vi "Test Draw Polylines ARGB.vi"(8 "error in (no error)":errorcluster, 11 "Test Case In":refnum<class "Image.lvclass">) -> (0 "error out":errorcluster, 3 "Test Case Out":refnum<class "Image.lvclass">)   [LabVIEW 2020, in "g_ar_toolkit.test.lvlib" / "Image.lvclass"]
uses:
  Image.lvclass
  C:/Program Files (x86)/National Instruments/LabVIEW 2020/vi.lib/Astemes/LUnit/Test Case.lvclass
  g_ar_toolkit.image/ARGB Colour.ctl
  g_ar_toolkit.common/Image Size (Integer).ctl
  g_ar_toolkit.common/Image Point (Integer).ctl
  <vilib>/Astemes/LUnit/Test Case.lvclass/Test Case.ctl
  g_ar_toolkit.image/CreateEmptyImageARGB.vi
  4993e8ee-a06a-463a-9684-69129f64d5ce.vi
  g_ar_toolkit.image/CreateEmptyImageARGB.vi/3321fa97-f432-4e1e-8db9-a0df79aed21b.vi
  g_ar_toolkit.image/DrawPolyLinesOnImageARGB.vi/f4fe866f-059f-471d-887d-2797bd4b3b13.vi
  g_ar_toolkit.image/DrawImageToPictureARGB.vi/8cd07b1b-062e-4fe4-9e87-2eb3dc89fe0e.vi
  <vilib>/Astemes/LUnit/Append Pass Result.vi
  <vilib>/Astemes/LUnit/Append Fail Result.vi
  <vilib>/Astemes/LUnit/Describe Comparison.vi
  <vilib>/Astemes/LUnit/Compare Variants.vi
  <vilib>/Astemes/LUnit/Run In UI.vi
  <vilib>/Utility/error.llb/Clear Errors.vi
  g_ar_toolkit.image/ARGBColourToU32.vi
  g_ar_toolkit.common/Module Path.vi
  <vilib>/Utility/error.llb/Error Cluster From Error Code.vi
  <vilib>/Astemes/LUnit/Describe Variant.vi
  Image.lvclass/Image.ctl
  g_ar_toolkit.image/g_ar_toolkit.image.lvlib
  g_ar_toolkit.common/g_ar_toolkit.common.lvlib
panel:
  out "Picture":picture
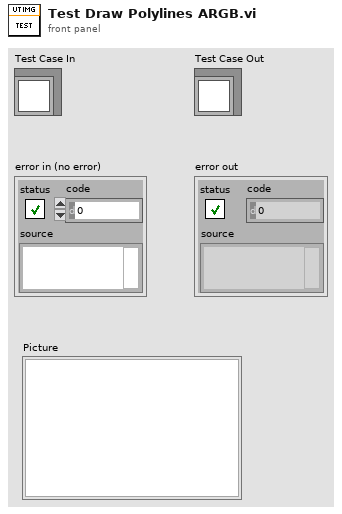
[diagram p1: front panel]
types:
  T1 = typedef "g_ar_toolkit.common.lvlib/Image Point (Integer).ctl" = cluster{"x":i32, "y":i32}
  T2 = typedef "g_ar_toolkit.image.lvlib/ARGB Colour.ctl" = cluster{"Alpha":u8, "RGB":u32}
  T3 = typedef "g_ar_toolkit.common.lvlib/Image Size (Integer).ctl" = cluster{"Width":u16, "Height":u16}
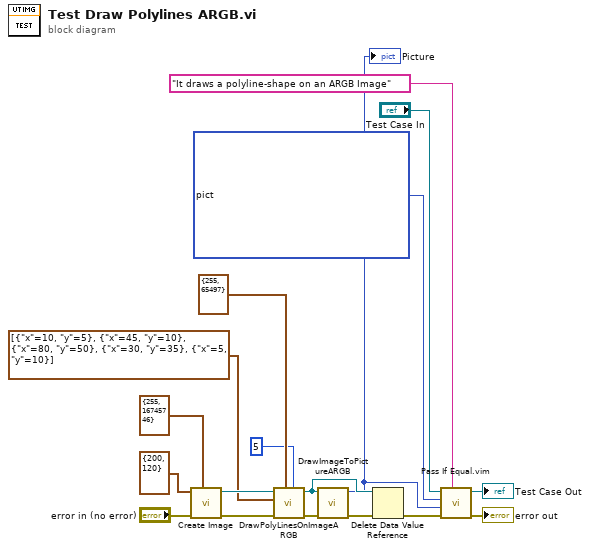
[diagram p0: block diagram]
diagram:
  n1 = call-poly "Create Image.vi"("Colour (Default: Black)"=T2 {"Alpha"=255, "RGB"=16745746}, "error in (no error)"="error in (no error)", "Preallocated Image Size (Default: 0,0)"=T3 {"Width"=200, "Height"=120}) -> ("error out"=w11:errorcluster, "New ARGB Image"=w12:refnum<data-value>)  [unwired: 7 in]
  n2 = call "DrawPolyLinesOnImageARGB.vi"("Thickness (Default: 1)"=u16 5, "ARGB Colour"=T2 {"Alpha"=255, "RGB"=65497}, "error in (no error)"=w11, "Points"=T1[] [{"x"=10, "y"=5}, {"x"=45, "y"=10}, {"x"=80, "y"=50}, {"x"=30, "y"=35}, {"x"=5, "y"=10}] ("Array"), "ARGB Image"=w12) -> ("error out"=w9:errorcluster, "ARGB Image (Duplicate)"=w10:refnum<data-value>)  [unwired: 5 in]
  n3 = call "DrawImageToPictureARGB.vi"("error in (no error)"=w9, "ARGB Image Source"=w10) -> ("error out"=w8:errorcluster, "Picture"=w5:picture)  [unwired: 8 in]
  "Picture" <- w5
  n4 = Delete Data Value Reference(data value reference=w10, error in=w8) -> (error out=w14:errorcluster)  [unwired: 1 out]
  n5 = call "Pass If Equal.vim"("Description"="It draws a polyline-shape on an ARGB Image", "error in (no error)"=w14, "Actual"=w5, "Expected"=picture bytes[72030] ("Picture"), "LUnit Test Case In"="Test Case In") -> ("error out"=→"error out":errorcluster, "LUnit Test Case Out"=→"Test Case Out":refnum<class "Image.lvclass">)  [unwired: 5 in]
